vi "visible_sub_vi.vi"() -> ()   [LabVIEW 2023]
panel:
  in  "Boolean":bool
  out "error out":errorcluster
  in  "error in (no error)":errorcluster
  in  "Ctl Refnum":refnum<vi>
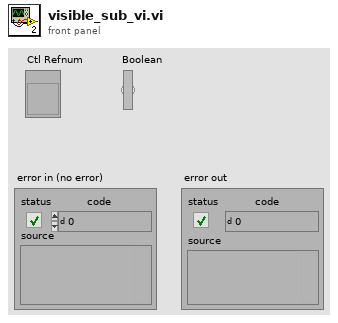
[diagram p1: front panel]
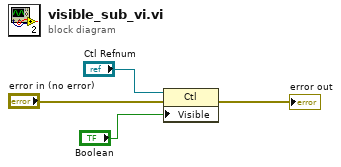
[diagram p0: block diagram]
diagram:
  n1 = property class="Ctl"(reference="Ctl Refnum", error in="error in (no error)", "Visible"="Boolean") -> (error out=→"error out":errorcluster)  [unwired: 1 out]
